vi "DFD I8 to FXP (vector).vi"(7 "quantization settings":T1={"source"=0, "wl"=16, "iwl"=1, "overflow mode"=enum."Wrap", "rounding mode"=enum."Truncation", "signed?"=TRUE} {"source" items=["Coefficients a/k"=0, "Coefficients b/v"=7, "Input"=1, "Output"=2, "Multiplicand"=3, "Product"=4, "Sum"=5, "Delay"=6]}, 8 "error in (no error)":errorcluster, 11 "I8 values":i8[](array[numeric])) -> (0 "error out":errorcluster, 3 "FXP values":dbl[](array[numeric]))   [LabVIEW 2017, in "NI_DigFilterLicensed.lvlib"]
doc: "Converts integers to fixed-point numbers. Wire data to the <B>I16</B> input to determine the polymorphic instance to use or manually select the instance."
uses:
  <vilib>/addons/Digital Filter Design/NI_DigFilterLicensed.lvlib
  <vilib>/addons/Digital Filter Design/_Objects.llb/DFD Quantization Settings.ctl
  <vilib>/addons/Digital Filter Design/_Objects.llb/DFD Quantization Sources.ctl
  <vilib>/addons/Digital Filter Design/FXPLib.llb/dfd_FXP Casting (vector).vi
  <vilib>/addons/Digital Filter Design/NI_DigFilter_FXP.lvlib
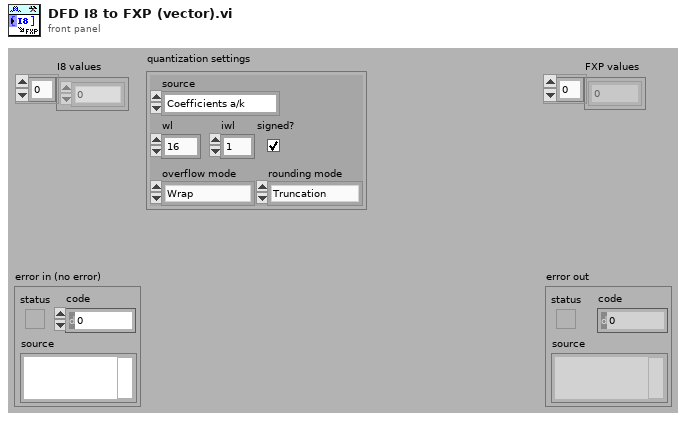
[diagram p1: front panel]
types:
  T1 = typedef "NI_DigFilterLicensed.lvlib/DFD Quantization Settings.ctl" = cluster{"source":T2, "wl":i16, "iwl":i16, "overflow mode":enum16{"Saturation", "Wrap"}, "rounding mode":enum16{"Nearest", "Truncation"}, "signed?":bool}
  T2 = typedef "NI_DigFilterLicensed.lvlib/DFD Quantization Sources.ctl" = u16
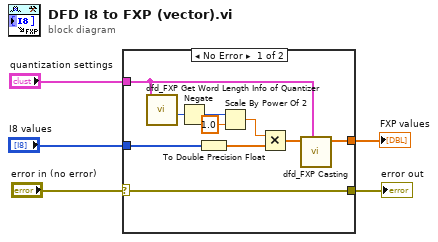
[diagram p0: block diagram]
diagram:
  n1 = case shown="No Error" "error in (no error)" {
    selector: "error in (no error)" -> [w6 w16]
    tunnel: "I8 values" -> [w13 _]
    tunnel: [w10 _] -> w4
    tunnel: "quantization settings" -> [w9 _]
    tunnel: [w6 w16] -> w1
    frame No Error {
      n2 = call <vilib>:"dfd_FXP Get Word Length Info of Quantizer.vi"("quantization settings"=w9) -> ("fwl"=w15:i16)  [unwired: 10 out]
      n3 = Negate(x=w15) -> (-x=w12:i16)
      n4 = To Double Precision Float(number=w13) -> (double precision float=w7:dbl[])
      n5 = Scale By Power Of 2(n=w12, x=1.0) -> (x*2^n=w8:dbl)
      n6 = Multiply(x=w8, y=w7) -> (x*y=w11:dbl[])
      n7 = call-poly <vilib>:"dfd_FXP Casting.vi"("quantization settings"=w9, "values in"=w11) -> ("values out"=w10:dbl[])  [unwired: 1 in, 6 out]
    }
    frame Error {
    }
  }
  "FXP values" <- w4
  "error out" <- w1
